vi "ctrlDP.vi"(0 "x":dbl, 1 "y":dbl, 2 "psi":dbl, 3 "PID 0":T1={"proportional gain (Kc)"=0.5, "integral time (Ti, min)"=0.0, "derivative time (Td, min)"=0.0}, 4 "PID 1":T1={"proportional gain (Kc)"=0.5, "integral time (Ti, min)"=0.0, "derivative time (Td, min)"=0.0}, 5 "PID 2":T1={"proportional gain (Kc)"=0.5, "integral time (Ti, min)"=0.0, "derivative time (Td, min)"=0.0}) -> (9 "psiplot":cluster{"Double":dbl, "y_r":dbl, "y":dbl}, 11 "yplot":cluster{"Double":dbl, "y_r":dbl, "y":dbl}, 13 "xplot":cluster{"Double":dbl, "y_r":dbl, "y":dbl}, 14 "u_0":dbl, 15 "u_1":dbl, 16 "u_2":dbl, 17 "eta_e_n":dbl[](array[numeric]), 18 "eta_e_b":dbl[](array[numeric]))   [LabVIEW 2014]
uses:
  <vilib>/Simulation/Scripting/Companion Diagram/SimConfigNode/SimParams.ctl
  <vilib>/Simulation/Scripting/Companion Diagram/SimConfigNode/_simSolvers.ctl
  <vilib>/Simulation/Implementation/Shared/SIMSCR Execution Mode.ctl
  <vilib>/Simulation/Param Hierarchy/Typedefs/SIMPH Param Control Actions.ctl
  <vilib>/Simulation/Implementation/Shared/NILVSim_ParamChanged.vi
  <vilib>/Simulation/Implementation/Shared/NILVSIM_BeginStep.vi
  <vilib>/Simulation/Implementation/Shared/NILVSim_Manager.vi
  <vilib>/Utility/error.llb/Clear Errors.vi
  <vilib>/Simulation/Implementation/Shared/NILVSim_FinalizeModel.vi
  <vilib>/Simulation/Implementation/Shared/SIM Unbundle Sim Info.vi
  <vilib>/Simulation/Implementation/Shared/NILVSim_Initialize.vi
  <vilib>/Simulation/Utility/Implementation/NILVSim Get Time and IsAcceptedStep.vi
  <vilib>/Simulation/Implementation/Shared/SIMSH Read Queue.vi
  <vilib>/Simulation/Implementation/Shared/NILVSim_GetModelError.vi
  <vilib>/Simulation/Implementation/Shared/SIM Bundle Sim Info.vi
  <vilib>/imath/engines/lvmath2/RunTimeEngine/NodeEndStatement/NIMS_NodeEndStatement_Output.vi
  <instcachedir>/0/NIMS_NodeEndStatement_Output_53EC0D466D134D7ABD903AC30B43404B.lvgen/NIMS_NodeEndStatement_Output_53EC0D466D134D7ABD903AC30B43404B_001.vi
  <vilib>/imath/engines/lvmath2/RunTimeEngine/ErrorHandling/NIMS_Finalize Error.vi
  <vilib>/addons/control/pid/pid.llb/PID (DBL).vi
  <vilib>/Simulation/Implementation/XNodeFramework/SimXNode/SimX.xnode
  subVIs/refModelDP3rd.vi
  <vilib>/Simulation/Scripting/Companion Diagram/SimConfigNode/SimDog.xnode
  <vilib>/addons/control/pid/NI_PID_pid.lvlib
  <vilib>/Simulation/Implementation/Shared/NI_SIM_Implementation.lvlib
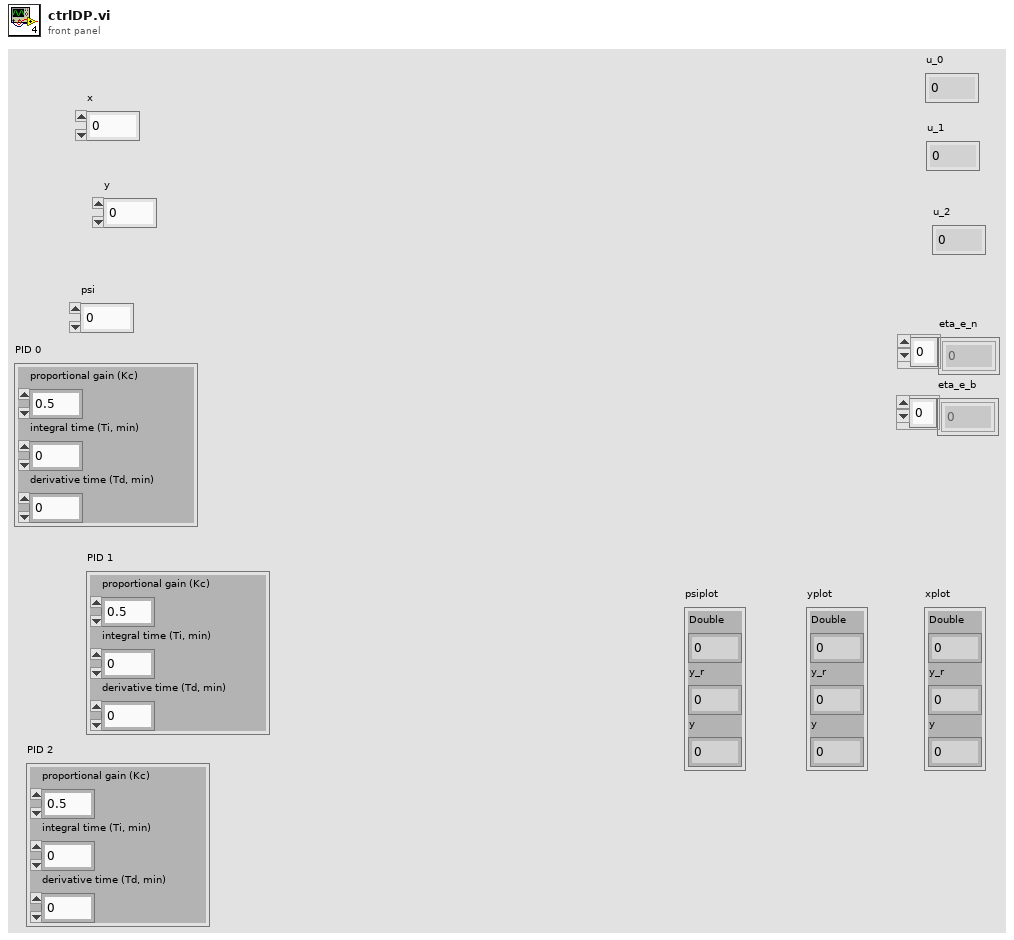
[diagram p1: front panel]
types:
  T1 = cluster{"proportional gain (Kc)":dbl, "integral time (Ti, min)":dbl, "derivative time (Td, min)":dbl}
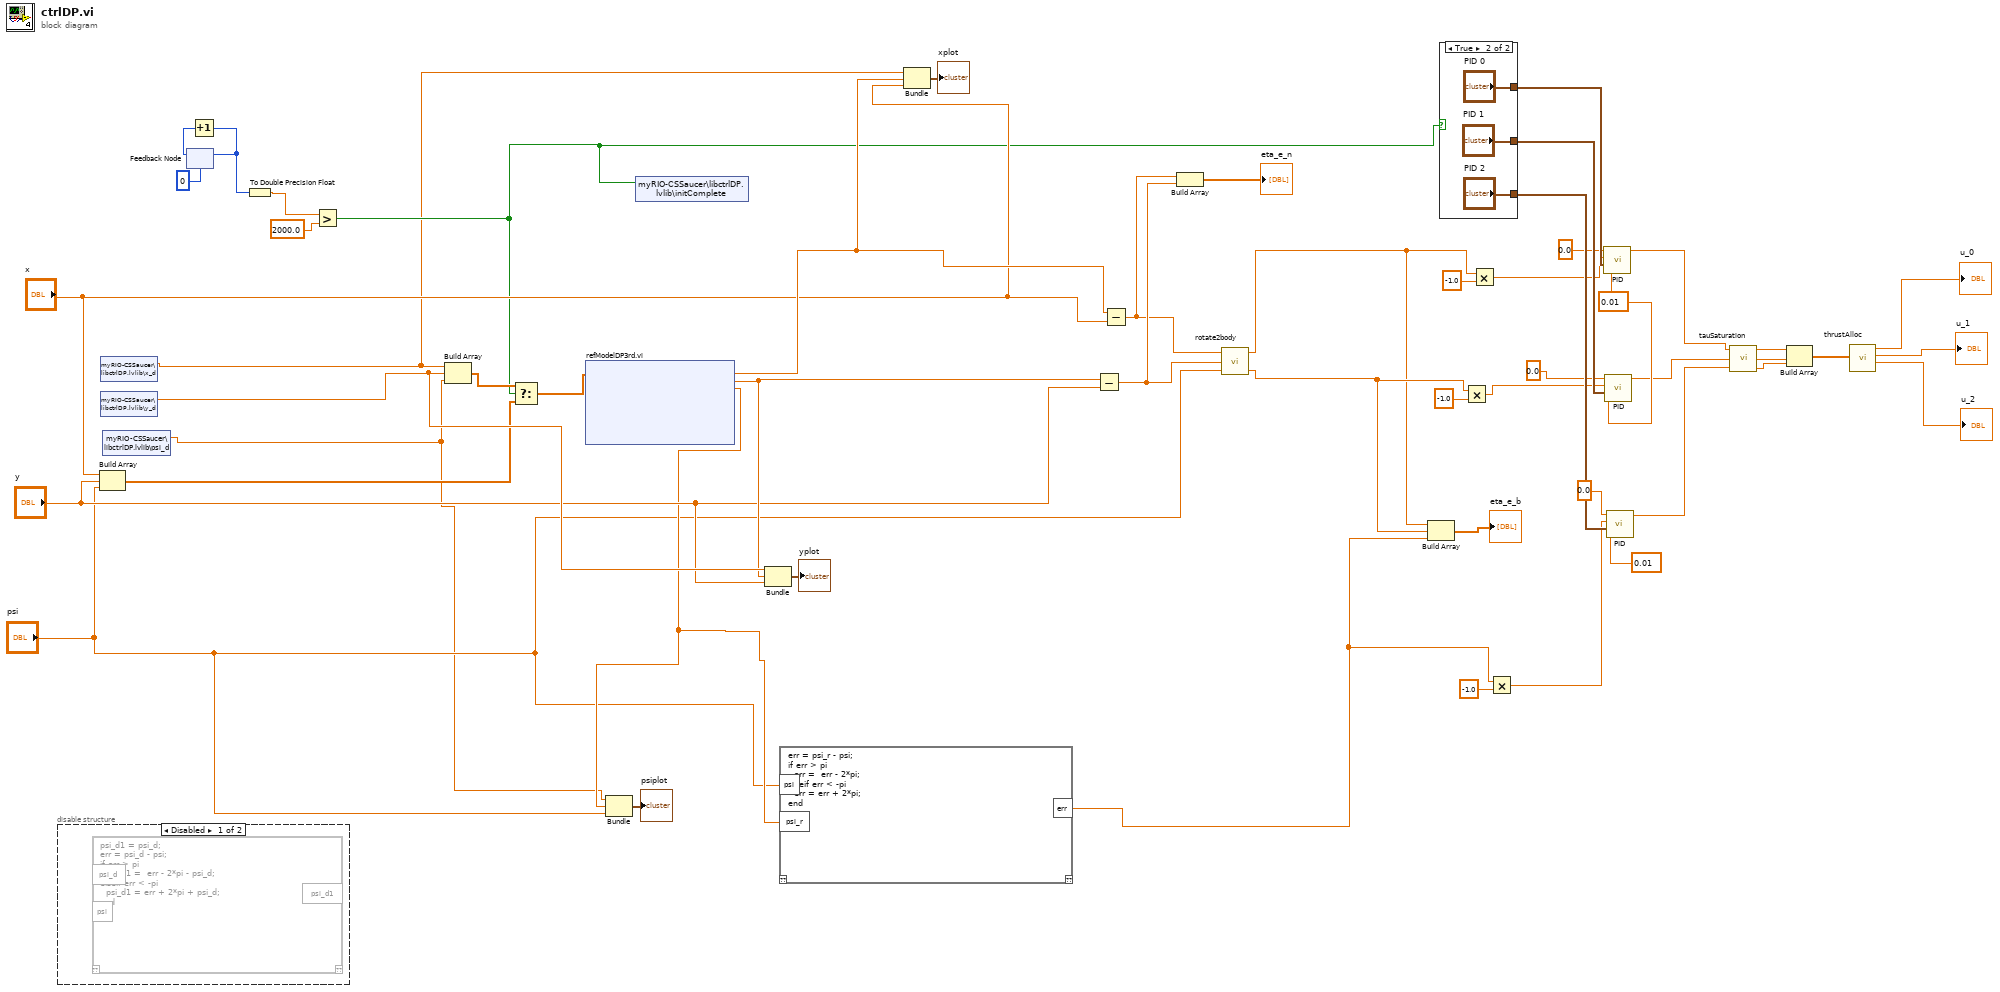
[diagram p0: block diagram]
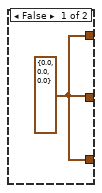
[diagram p3: hidden frame]
diagram:
  w52 = 0.01 ("dt (s)")
  n1 = disable-structure shown="Disabled" {
    frame Disabled {
      n2 = mathscript code="psi_d1 = psi_d;\nerr = psi_d - psi;\nif err > pi\n  psi_d1 =  err - 2*pi - psi_d;\nelseif err < -pi\n  psi_d1 = err + 2*pi + psi_d;\nend"() -> ()  [unwired: 3 in, 2 out]
    }
    frame Enabled {
    }
  }
  n3 = Build Array("x", "y", "psi") -> (w12:dbl[])
  n4 = shared-variable "myRIO-CSSaucer\\libctrlDP.lvlib\\x_d"() -> (w5:dbl)  [unwired: 1 in, 1 out]
  n5 = shared-variable "myRIO-CSSaucer\\libctrlDP.lvlib\\y_d"() -> (w39:dbl)  [unwired: 1 in, 1 out]
  n6 = shared-variable "myRIO-CSSaucer\\libctrlDP.lvlib\\psi_d"() -> (w1:dbl)  [unwired: 1 in, 1 out]
  n7 = feedback #1(u32 0 ("f")) -> (w8:u32)
  n8 = Increment(x=w8) -> (x+1=w6:u32)
  n9 = feedback-in #1(w6) -> ()
  n10 = To Double Precision Float(number=w6) -> (double precision float=w7:dbl)
  n11 = Greater?(x=w7, y=2000.0) -> (0:w10:bool)
  n12 = Build Array(w5, w39, w1) -> (w13:dbl[])
  n13 = Select(t=w13, s=w10, f=w12) -> (s? t:f=w11:dbl[])
  n14 = xnode "refModelDP3rd.vi"("eta_d"=w11) -> ("x_r"=w24:dbl, "y_r"=w23:dbl, "psi_r"=w4:dbl)  [unwired: 2 in, 9 out]
  n15 = Bundle("Double"=w1, "psi_r"=w4, "psi"="psi") -> (→"psiplot":cluster{"Double":dbl, "psi_r":dbl, "psi":dbl})  [unwired: 1 in]
  n16 = shared-variable "myRIO-CSSaucer\\libctrlDP.lvlib\\initComplete"(w10) -> ()  [unwired: 1 in, 1 out]
  n17 = Bundle("Double"=w39, "y_r"=w23, "y"="y") -> (→"yplot":cluster{"Double":dbl, "y_r":dbl, "y":dbl})  [unwired: 1 in]
  n18 = mathscript code="err = psi_r - psi;\nif err > pi\n  err =  err - 2*pi;\nelseif err < -pi\n  err = err + 2*pi;\nend"("psi"="psi", "psi_r"=w4) -> ("err"=w3:dbl)  [unwired: 1 in, 1 out]
  n19 = Bundle("Double"=w5, "x_r"=w24, "x"="x") -> (→"xplot":cluster{"Double":dbl, "x_r":dbl, "x":dbl})  [unwired: 1 in]
  n20 = Subtract(x=w23, y="y") -> (x-y=w42:dbl)
  n21 = Subtract(x=w24, y="x") -> (x-y=w41:dbl)
  n22 = Build Array(w41, w42) -> (→"eta_e_n":dbl[])
  n23 = call "rotate2body.vi"("psi"="psi", "2"=w42, "1"=w41) -> ("2_body"=w34:dbl, "1_body"=w29:dbl)  [unwired: 1 in]
  n24 = Build Array(w29, w34, w3) -> (→"eta_e_b":dbl[])
  n25 = case shown="True" w10 {
    tunnel: [w131 "PID 0"] -> w46
    tunnel: [w131 "PID 1"] -> w45
    tunnel: [w131 "PID 2"] -> w44
    frame False {
      w131 = T1 {"proportional gain (Kc)"=0.0, "integral time (Ti, min)"=0.0, "derivative time (Td, min)"=0.0} ("PID 0")
    }
    frame True {
    }
  }
  n26 = Multiply(x=w34, y=-1.0) -> (x*y=w33:dbl)
  n27 = Multiply(x=w29, y=-1.0) -> (x*y=w27:dbl)
  n28 = Multiply(x=w3, y=-1.0) -> (x*y=w25:dbl)
  n29 = call-poly <vilib>:"PID.vi"("dt (s)"=w52, "PID gains"=w46, "process variable"=w27, "setpoint"=0.0 ("process variable")) -> ("output"=w18:dbl)  [unwired: 6 in, 1 out]
  n30 = call-poly <vilib>:"PID.vi"("dt (s)"=w52, "PID gains"=w45, "process variable"=w33, "setpoint"=0.0 ("process variable")) -> ("output"=w19:dbl)  [unwired: 6 in, 1 out]
  n31 = call-poly <vilib>:"PID.vi"("dt (s)"=0.01, "PID gains"=w44, "process variable"=w25, "setpoint"=0.0 ("process variable")) -> ("output"=w20:dbl)  [unwired: 6 in, 1 out]
  n32 = call "tauSaturation.vi"("N"=w20, "Y"=w19, "X"=w18) -> ("Nout"=w15:dbl, "Yout"=w16:dbl, "Xout"=w17:dbl)
  n33 = Build Array(w17, w16, w15) -> (w50:dbl[])
  n34 = call "thrustAlloc.vi"("tau"=w50) -> ("u_0"=→"u_0":dbl, "u_1"=→"u_1":dbl, "u_2"=→"u_2":dbl)  [unwired: 5 in]
